vi "RSZVB Set Source Power Calibration Port State.vi"(7 "Port State (F: Off)":bool, 8 "error in (no error)":errorcluster {"code" format="%.0x"}, 9 "Port Number (1)":i32=1, 10 "Channel (1)":i32=1, 11 "VISA session":refnum<visa-resource-name>) -> (0 "error out":errorcluster {"code" format="%.0x"}, 3 "dup VISA session":refnum<visa-resource-name>)   [LabVIEW 2011]
doc: "This VI enables or disables the source power calibration for channel <Ch> and for port number <Pt>. \n\nNotes:\n\n(1) The command is disabled unless a source power calibration for the analyzer port has been performed (rszvb_InitiateSourcePowerCalibration). \n\n(2) To enable or disable a source power calibration for an external generator use SOURce<Ch>:POWer<Pt>:CORRection:GENerator[:STATe].\n\nRemote-control command(s):\nSOURce<Ch>:POWer<Pt>:CORRection[:STATe] ON | OFF"
uses:
  _utility/RSZVB Global Data.vi
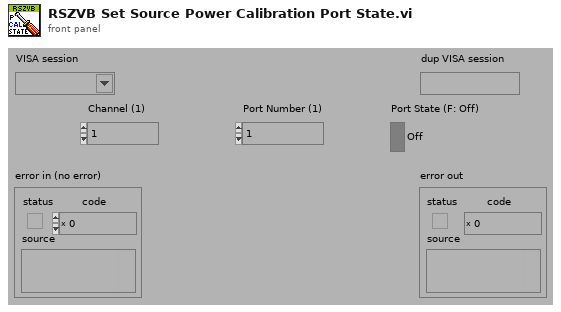
[diagram p1: front panel]
types:
  T1 = cluster{"Error Checking (T: On)":bool, "Installed Options":string[], "Data Valid?":bool, "Ports":i32, "Model":string[], "Option Checking (T: On)":bool}[]
  T2 = cluster{"Error Checking (T: On)":bool, "Installed Options":string[], "Data Valid?":bool, "Ports":i32, "Model":string[], "Option Checking (T: On)":bool}
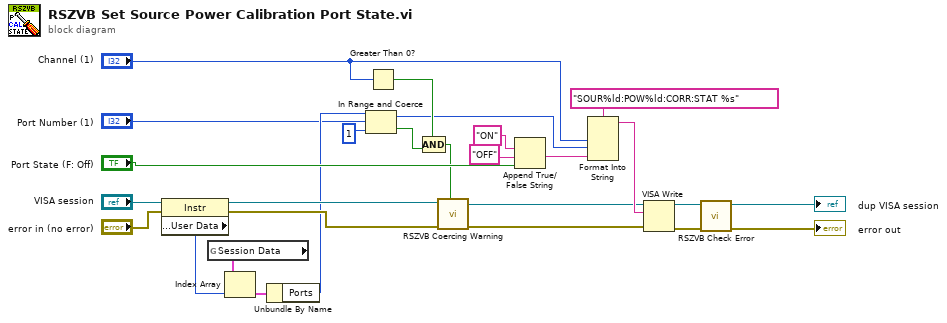
[diagram p0: block diagram]
diagram:
  n1 = property class="Instr"(reference="VISA session", error in="error in (no error)") -> (reference out=w11:refnum<visa-resource-name>, error out=w10:errorcluster, "General Settings:User Data"=w14:u32)
  n2 = global read "RSZVB Global Data.vi" "Session Data"() -> (w15:T1)
  n3 = Index Array(array=w15, index=w14) -> (element=w16:T2)
  n4 = Unbundle By Name(w16) -> ("Ports"=w5:i32)
  n5 = In Range and Coerce(upper limit=w5, x="Port Number (1)", lower limit=1) -> (coerced(x)=w1:i32, In Range?=w6:bool)
  n6 = Greater Than 0?(x="Channel (1)") -> (x > 0?=w2:bool)
  n7 = Compound Arithmetic op=AND(w2, w6) -> (w3:bool)
  n8 = call "RSZVB Coercing Warning.vi"("In Range?"=w3, "error in (no error)"=w10, "VISA session"=w11) -> ("error out"=w21:errorcluster, "dup VISA session"=w20:refnum<visa-resource-name>)  [unwired: 7 in]
  n9 = Append True/False String(1:"Port State (F: Off)", 2:"OFF", 3:"ON") -> (0:w19:string)  [unwired: 1 in]
  n10 = Format Into String(format string="SOUR%ld:POW%ld:CORR:STAT %s", "Channel (1)", w1, w19) -> (resulting string=w24:string)  [unwired: 2 in, 1 out]
  n11 = VISA Write(VISA resource name=w20, write buffer=w24, error in (no error)=w21) -> (VISA resource name out=w25:refnum<visa-resource-name>, error out=w26:errorcluster)  [unwired: 1 out]
  n12 = call "RSZVB Check Error.vi"("error in (no error)"=w26, "VISA session"=w25) -> ("error out"=→"error out":errorcluster, "dup VISA session"=→"dup VISA session":refnum<visa-resource-name>)  [unwired: 8 in]
